vi "Is Name valid Multiplatform.vi"(8 "error in (no error)":errorcluster caption="entrée d'erreur (pas d'erreur)", 10 "filename must be valid on all platforms (F)":bool caption="le nom de fichier doit être valide sur toutes les plates-formes (F)", 11 "filename":string caption="nom de fichier") -> (0 "error out":errorcluster caption="sortie d'erreur", 1 "filename not crossplatform":bool caption="nom de fichier non multiplate-forme", 2 "filename had conflict":bool caption="conflit de nom de fichier", 3 "suggested filename":string caption="nom de fichier suggéré", 4 "problem description":string caption="description du problème")   [LabVIEW 2019]
doc: "Vérifie si un nom de fichier est valide sur différentes plates-formes. Ce VI vérifie le nom des fichiers pour les plates-formes qui supportent LabVIEW, autrement dit Windows, OS X et Linux. Vous pouvez choisir de vérifier le nom de fichier pour toutes les plates-formes ou la plate-forme actuelle."
panel:
  in  "Platform Warnings":string[](array[string])=["Les noms de fichiers Windows ne peuvent contenir aucun des caractères : \\ : / * ? \" < > |.", "Les noms de fichiers Windows ne peuvent pas se terminer par un point.", "Les noms de fichiers Macintosh ne peuvent pas contenir le caractère :.", "Les noms de fichiers Linux ne peuvent pas contenir le caractère /."] caption="Mises en garde de plate-forme"
  in  "Empty filename":string="Une chaîne vide n'est pas un nom de fichier valide." caption="Nom de fichier vide"
  in  "Contains Multibyte":string="%s contient des caractères multi-octets." caption="Contient des car. multioctets"
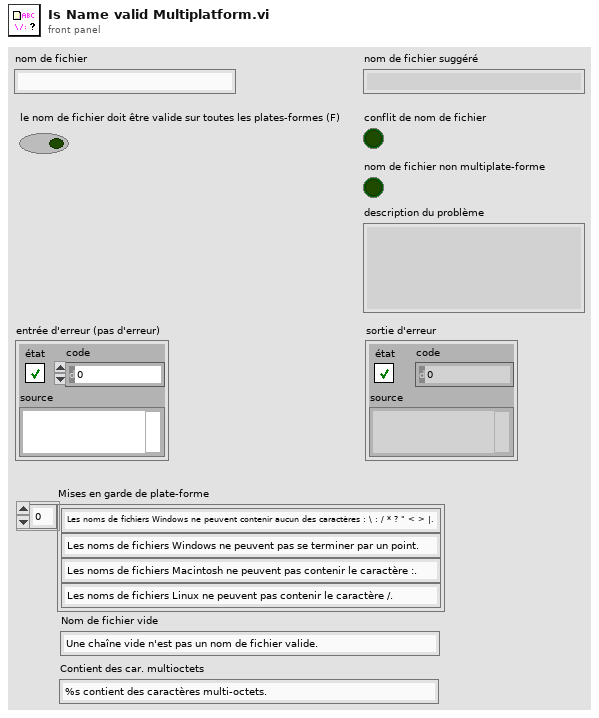
[diagram p1: front panel]
types:
  T1 = cluster{enum32{"invalid OS target", "Mac OS", "Windows 3.1", "Windows 95/NT", "Solaris 1", "Solaris 2", "HP-UX", "PowerMAX", "Linux", "Irix", "Rhapsody", "BeOS", "AIX", "OSF1", "VxWorks", "PharLap", "Carbon", "RTX", "Windows x64", "Linux x64", "Mac OS X x64"}[]}[]
  T2 = enum32{"invalid OS target", "Mac OS", "Windows 3.1", "Windows 95/NT", "Solaris 1", "Solaris 2", "HP-UX", "PowerMAX", "Linux", "Irix", "Rhapsody", "BeOS", "AIX", "OSF1", "VxWorks", "PharLap", "Carbon", "RTX", "Windows x64", "Linux x64", "Mac OS X x64"}
  T3 = enum32{"invalid OS target", "Mac OS", "Windows 3.1", "Windows 95/NT", "Solaris 1", "Solaris 2", "HP-UX", "PowerMAX", "Linux", "Irix", "Rhapsody", "BeOS", "AIX", "OSF1", "VxWorks", "PharLap", "Carbon", "RTX", "Windows x64", "Linux x64", "Mac OS X x64"}[]
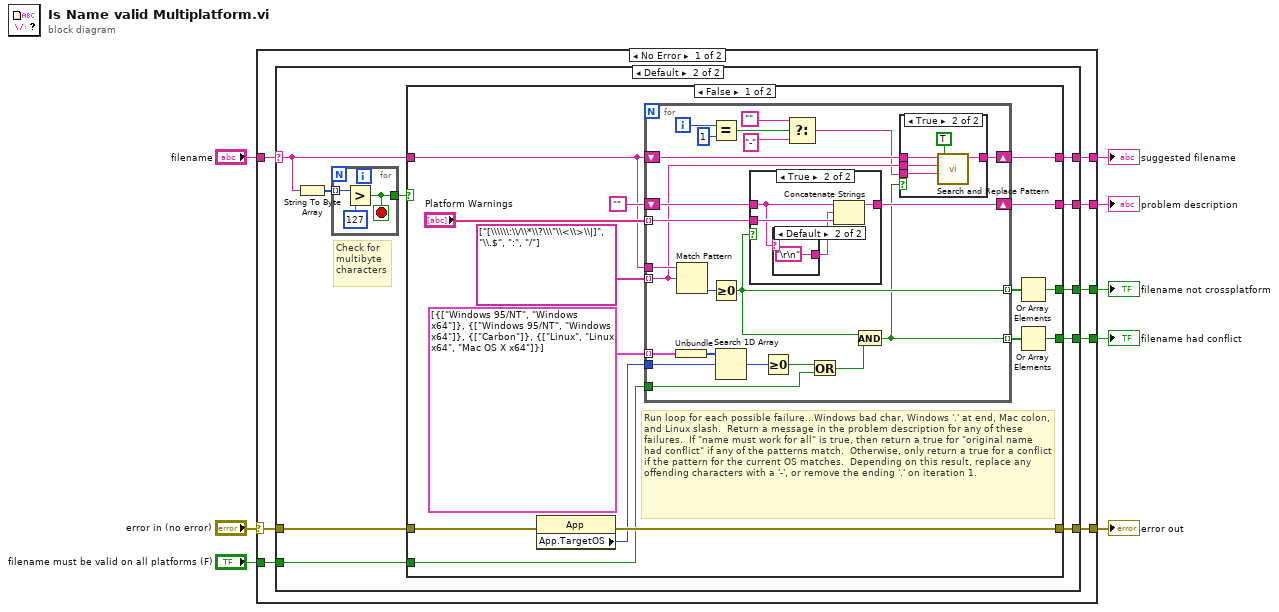
[diagram p0: block diagram]
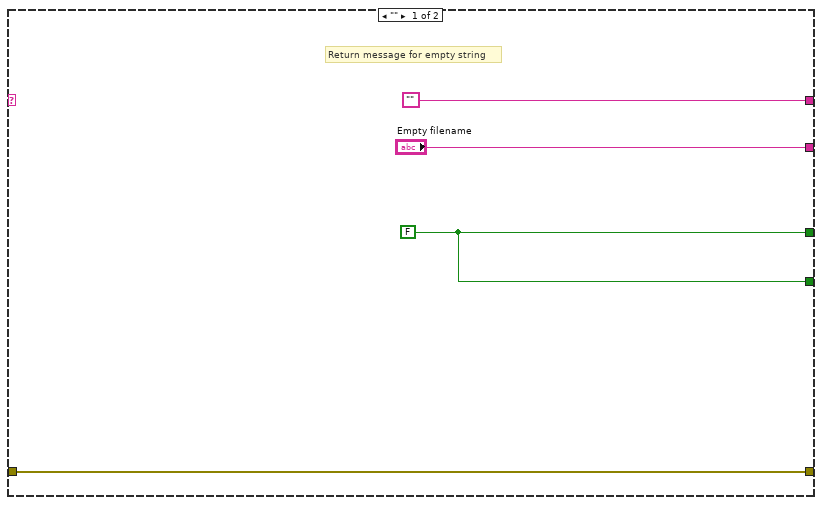
[diagram p2: hidden frame]
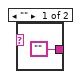
[diagram p5: hidden frame]
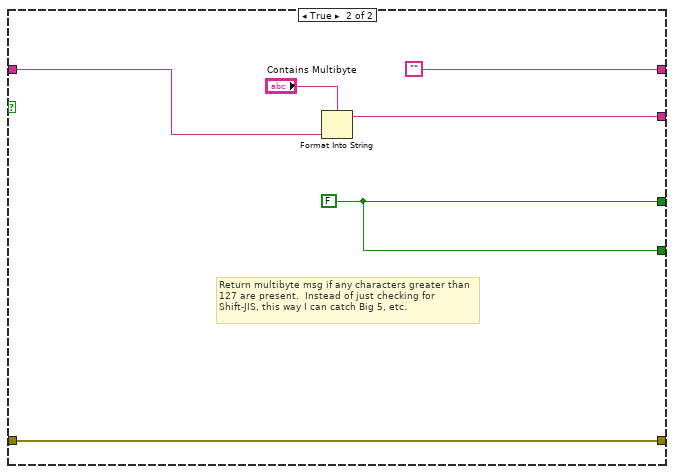
[diagram p6: hidden frame]
diagram:
  n1 = case shown="No Error" "error in (no error)" {
    selector: "error in (no error)" -> [w9 w91]
    tunnel: [w16 _] -> w8
    tunnel: [w15 _] -> w7
    tunnel: [w14 _] -> w6
    tunnel: [w13 _] -> w5
    tunnel: "filename" -> [w12 _]
    tunnel: "filename must be valid on all platforms (F)" -> [w11 _]
    tunnel: [w10 w91] -> w1
    frame No Error {
      n2 = case shown="Default" w12 {
        selector: w12 -> [_ w26]
        tunnel: [w19 w30] -> w16
        tunnel: [w19 w29] -> w15
        tunnel: ["Empty filename" w28] -> w14
        tunnel: ["" w27] -> w13
        tunnel: w11 -> [_ w25]
        tunnel: [w18 w24] -> w10
        tunnel: w9 -> [w18 w23]
        frame "" {
          w19 = FALSE
          # "Return message for empty string"
        }
        frame Default {
          # "Check for\nmultibyte\ncharacters"
          n3 = String To Byte Array(string=w26) -> (unsigned byte array=w22:u8[])
          n4 = for {
            tunnel: w22 -> [w33] mode=indexing
            tunnel: [w31] -> w21
            stop <- w31 stop-if-true
            n5 = Greater?(x=w33, y=u8 127) -> (0:w31:bool)
          }
          n6 = case shown="False" w21 {
            tunnel: [w42 w86] -> w30
            tunnel: [w38 w86] -> w29
            tunnel: [w45 w89] -> w28
            tunnel: [w35 ""] -> w27
            tunnel: w26 -> [w36 w88]
            tunnel: w25 -> [w39 _]
            tunnel: [w41 w85] -> w24
            tunnel: w23 -> [w40 w85]
            frame False {
              # "Run loop for each possible failure...Windows bad char, Windows '.' at end, Mac colon, and Linux slash.  Return a message in the problem description for any of these failures.  If \"name must work for all\" is true, then return a true for \"original name had conflict\" if any of the patterns match.  Otherwise, only return a true for a conflict if the pattern for the current OS matches.  Depending on this result, replace any offending characters with a '-', or remove the ending '.' on iteration 1."
              n7 = property class="App"(error in=w40) -> (error out=w41:errorcluster, "App.TargetOS"=w34:T2)  [unwired: 1 in, 1 out]
              n8 = for {
                tunnel: string[] ["[\\\\\\:\\/\\*\\?\\\"\\<\\>\\|]", "\\.$", ":", "/"] -> [w55] mode=indexing
                tunnel: w36 -> [w70]
                shift-right: [w67] -> w45
                shift-left: "" -> [w69]
                tunnel: "Platform Warnings" -> [w68] mode=indexing
                tunnel: T1 [{[enum."Windows 95/NT", enum."Windows x64"]}, {[enum."Windows 95/NT", enum."Windows x64"]}, {[enum."Carbon"]}, {[enum."Linux", enum."Linux x64", enum."Mac OS X x64"]}] -> [w66] mode=indexing
                tunnel: w34 -> [w64]
                tunnel: [w62] -> w43 mode=indexing
                tunnel: w39 -> [w60]
                tunnel: [w56] -> w37 mode=indexing
                shift-right: [w57] -> w35
                shift-left: w36 -> [w58]
                i -> [w54]
                n9 = Unbundle(w66) -> (w65:T3)
                n10 = Match Pattern(string=w70, regular expression=w55) -> (offset past match=w71:i32)  [unwired: 4 out]
                n11 = Equal?(x=w54, y=1) -> (x = y?=w52:bool)
                n12 = Greater Or Equal To 0?(x=w71) -> (x >= 0?=w62:bool)
                n13 = Search 1D Array(1D array=w65, element=w64) -> (index of element=w63:i32)  [unwired: 1 out]
                n14 = case shown="True" w62 {
                  tunnel: w69 -> [w78 w80]
                  tunnel: w68 -> [_ w81]
                  tunnel: [w78 w82] -> w67
                  frame False {
                  }
                  frame True {
                    n15 = case shown="Default" w80 {
                      tunnel: ["" "\r\n"] -> w79
                      frame "" {
                      }
                      frame Default {
                      }
                    }
                    n16 = Concatenate Strings(w80, w79, w81) -> (w82:string)
                  }
                }
                n17 = Greater Or Equal To 0?(x=w63) -> (x >= 0?=w61:bool)
                n18 = Select(t="", s=w52, f="-" ("replace string (\"\")")) -> (s? t:f=w49:string)
                n19 = Or(x=w61, y=w60) -> (x .or. y?=w59:bool)
                n20 = And(x=w62, y=w59) -> (x .and. y?=w56:bool)
                n21 = case shown="True" w56 {
                  tunnel: w58 -> [w72 w77]
                  tunnel: [w72 w75] -> w57
                  tunnel: w55 -> [_ w74]
                  tunnel: w49 -> [_ w73]
                  frame False {
                  }
                  frame True {
                    n22 = call <vilib>:"Search and Replace Pattern.vi"("string"=w77, "regular expression (\"\")"=w74, "replace string (\"\")"=w73, "replace all? (F)"=TRUE) -> ("result string"=w75:string)  [unwired: 2 out]
                  }
                }
              }
              n23 = Or Array Elements(Boolean array=w43) -> (logical OR=w42:bool)
              n24 = Or Array Elements(Boolean array=w37) -> (logical OR=w38:bool)
            }
            frame True {
              w86 = FALSE
              # "Return multibyte msg if any characters greater than 127 are present.  Instead of just checking for Shift-JIS, this way I can catch Big 5, etc."
              n25 = Format Into String(format string="Contains Multibyte", w88) -> (resulting string=w89:string)  [unwired: 2 in, 1 out]
            }
          }
        }
      }
    }
    frame Error {
    }
  }
  "problem description" <- w6
  "filename not crossplatform" <- w8
  "filename had conflict" <- w7
  "suggested filename" <- w5
  "error out" <- w1
